vi "Create Poll Source Code Cron String.vi"(11 "Source Code Poll":T1) -> (3 "String":string)   [LabVIEW 2014]
uses:
  Controls/Source Code Control Selection - STYP.ctl
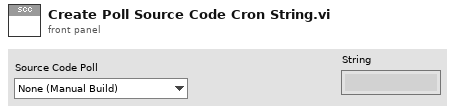
[diagram p1: front panel]
types:
  T1 = typedef "Source Code Control Selection - STYP.ctl" = enum16{"None (Manual Build)", "Every 15 Minutes", "Every 30 Minutes", "Every 45 Minutes", "Every Hour", "Every 2 Hours", "Everyday "}
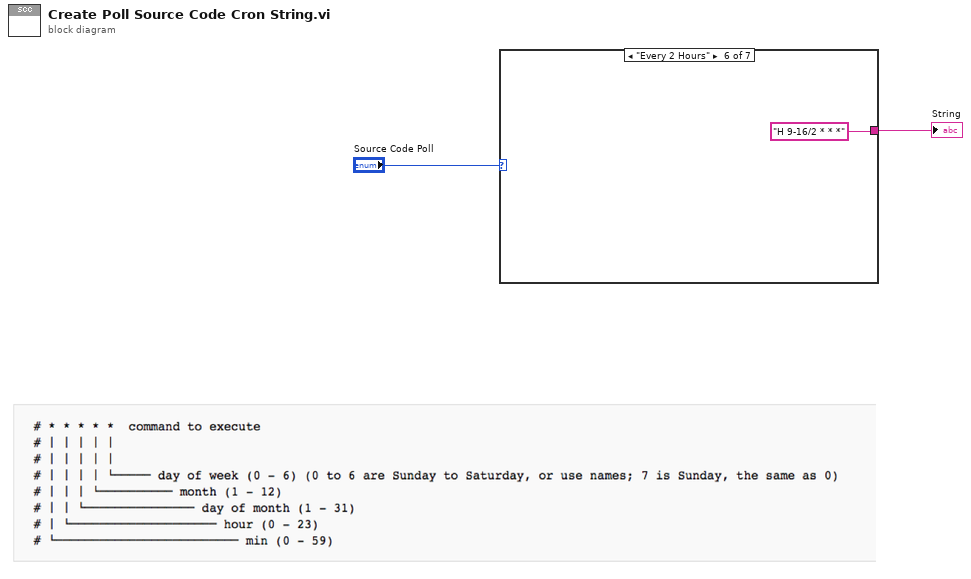
[diagram p0: block diagram]
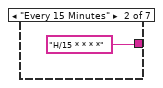
[diagram p3: hidden frame]
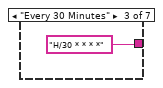
[diagram p4: hidden frame]
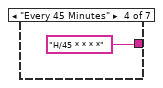
[diagram p5: hidden frame]
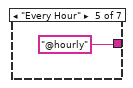
[diagram p6: hidden frame]
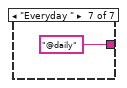
[diagram p7: hidden frame]
diagram:
  n1 = case shown="\"Every 2 Hours\"" "Source Code Poll" {
    tunnel: [_ "H/15 * * * *" ("format string") "H/30 * * * *" ("format string") "H/45 * * * *" ("format string") "@hourly" ("format string") "H 9-16/2 * * *" ("format string") "@daily" ("format string")] -> w2
    frame "None (Manual Build)", Default {
    }
    frame "Every 15 Minutes" {
    }
    frame "Every 30 Minutes" {
    }
    frame "Every 45 Minutes" {
    }
    frame "Every Hour" {
    }
    frame "Every 2 Hours" {
    }
    frame "Everyday " {
    }
  }
  "String" <- w2
